vi "parse.creators.vi"(7 "body":string, 8 "error in (no error)":errorcluster, 11 "issue_class in":refnum<class "issue_class.lvclass">) -> (0 "error out":errorcluster, 3 "issue_class out":refnum<class "issue_class.lvclass">)   [LabVIEW 2024, in "issue_class.lvclass"]
uses:
  issue_class.lvclass
  issue_class.lvclass/issue_class.ctl
  definitions/creator.ctl
  <vilib>/Utility/error.llb/Trim Whitespace One-Sided.vi
  comic_class/comic_class.lvclass
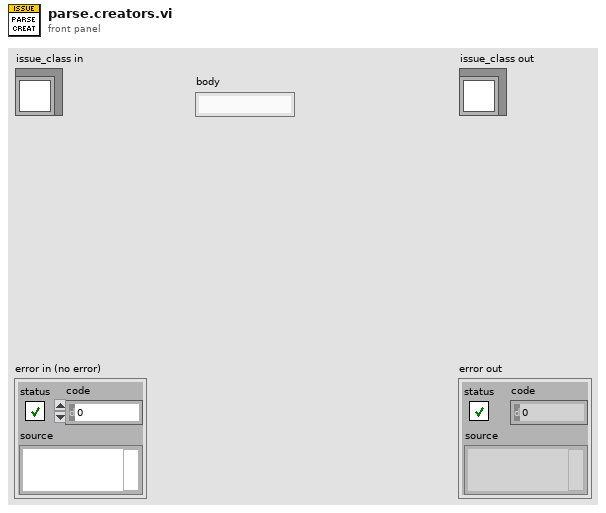
[diagram p1: front panel]
types:
  T1 = typedef "creator.ctl" = cluster{"name":string, "role":string, "url":string}
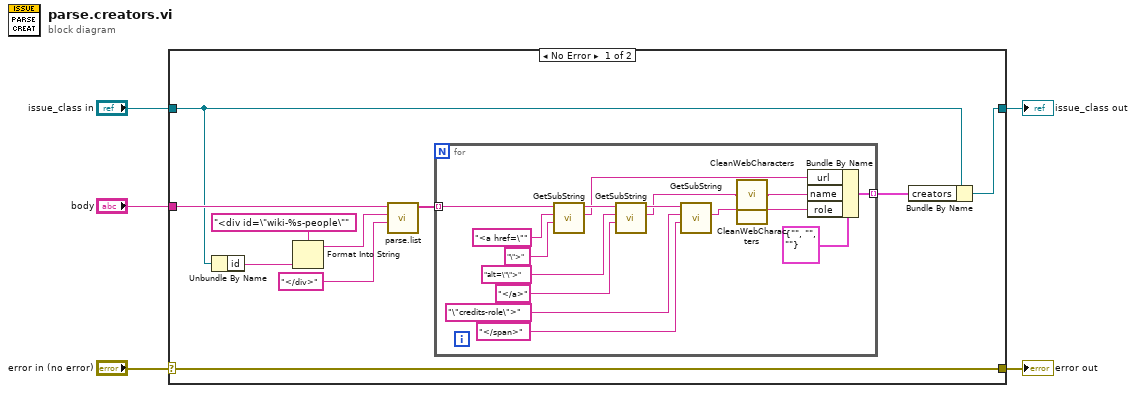
[diagram p0: block diagram]
diagram:
  n1 = case shown="No Error" "error in (no error)" {
    selector: "error in (no error)" -> [w15 w33]
    tunnel: [w15 w33] -> w4
    tunnel: [w7 w32] -> w2
    tunnel: "issue_class in" -> [w8 w32]
    tunnel: "body" -> [w14 _]
    frame No Error {
      n2 = Unbundle By Name(w8) -> ("id"=w13:string)
      n3 = Format Into String(format string="<div id=\"wiki-%s-people\"", w13) -> (resulting string=w11:string)  [unwired: 2 in, 1 out]
      n4 = call "parse.list.vi"("div end"="</div>", "div start"=w11, "body"=w14) -> ("list array"=w9:string[])  [unwired: 8 in]
      n5 = for {
        tunnel: w9 -> [w31] mode=indexing
        tunnel: [w20] -> w6 mode=indexing
        n6 = call "GetSubString.vi"("End Search"="\">", "Start Search"="<a href=\"" ("div end"), "String In"=w31) -> ("Match"=w21:string, "Following String Out"=w28:string)  [unwired: 6 in, 1 out]
        n7 = call "GetSubString.vi"("End Search"="</a>", "Start Search"="alt=\"\">" ("div end"), "String In"=w28) -> ("Match"=w17:string, "Following String Out"=w23:string)  [unwired: 6 in, 1 out]
        n8 = call "GetSubString.vi"("End Search"="</span>", "Start Search"="\"credits-role\">" ("div end"), "String In"=w23) -> ("Match"=w19:string)  [unwired: 6 in, 2 out]
        n9 = call "CleanWebCharacters.vi"("string in"=w17) -> ("string out"=w16:string)
        n10 = call "CleanWebCharacters.vi"("string in"=w19) -> ("string out"=w18:string)
        n11 = Bundle By Name(cluster=T1 {"name"="", "role"="", "url"=""} ("creator"), "url"=w21, "name"=w16, "role"=w18) -> (w20:T1)
      }
      n12 = Bundle By Name(cluster=w8, "creators"=w6) -> (w7:refnum<class "issue_class.lvclass">)
    }
    frame Error {
    }
  }
  "error out" <- w4
  "issue_class out" <- w2
